vi "get_size.vi"(8 "error in (no error)":errorcluster, 11 "HGF_FGV_Size":refnum<class "HGF_FGV_Size.lvclass">) -> (0 "error out":errorcluster, 2 "size":u32, 3 "HGF_FGV_Size":refnum<class "HGF_FGV_Size.lvclass">)   [LabVIEW 2012, in "HGF_FGV.lvlib" / "HGF_FGV_Size.lvclass"]
doc: "This VI returns the size of the object array stored in the FGV instance."
uses:
  HGF_FGV_Size.lvclass
  HGF_FGV_Size.lvclass/HGF_FGV_Size.ctl
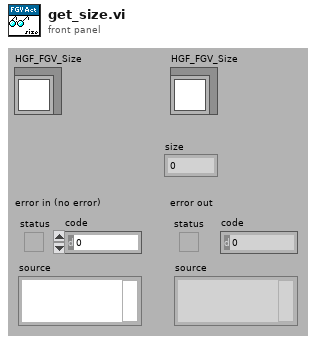
[diagram p1: front panel]
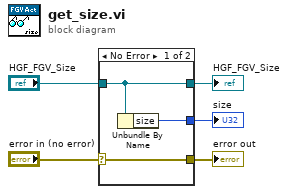
[diagram p0: block diagram]
diagram:
  n1 = case shown="No Error" "error in (no error)" {
    selector: "error in (no error)" -> [w8 w9]
    tunnel: [w8 w9] -> w4
    tunnel: [w7 w10] -> w2
    tunnel: "HGF_FGV_Size" -> [w7 w10]
    tunnel: [w6 _] -> w1
    frame No Error {
      n2 = Unbundle By Name(w7) -> ("size"=w6:u32)
    }
    frame Error {
    }
  }
  "error out" <- w4
  "HGF_FGV_Size" <- w2
  "size" <- w1
